vi "check syntax_core.vi"(8 "error in (no error)":errorcluster caption="에러 입력(에러 없음)", 11 "Script Line_gpio 입력":refnum<class "Script Line_gpio.lvclass">) -> (0 "error out":errorcluster caption="에러 출력", 3 "Script Line_gpio 출력":refnum<class "Script Line_gpio.lvclass">)   [LabVIEW 2020, in "Script Line_gpio.lvclass"]
uses:
  Script Line_gpio.lvclass
  Script Line/Script Line.lvclass/Script Line.ctl
  Script Line_gpio.lvclass/Script Line_gpio.ctl
  327cb276-063d-4ad0-890d-a8e0501d4965.vi
  Script Line/Accessors/Read parameter.vi
  Script Line/Accessors/Read parameter string index.vi
  <vilib>/Comparison/Equal/Equal Functor/Equal Functor.lvclass
  Script Line/Script Line.lvclass
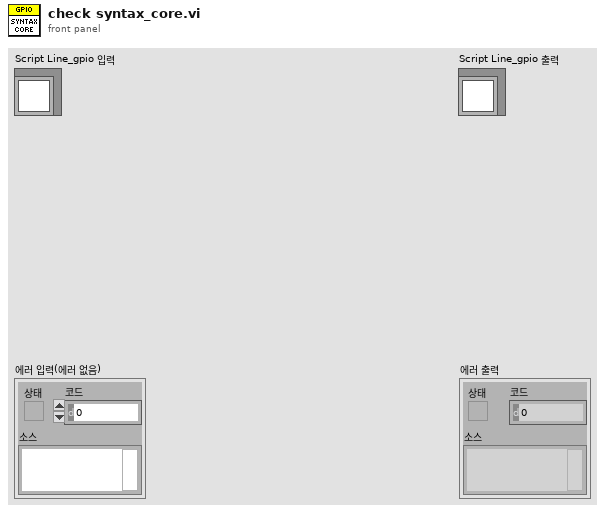
[diagram p1: front panel]
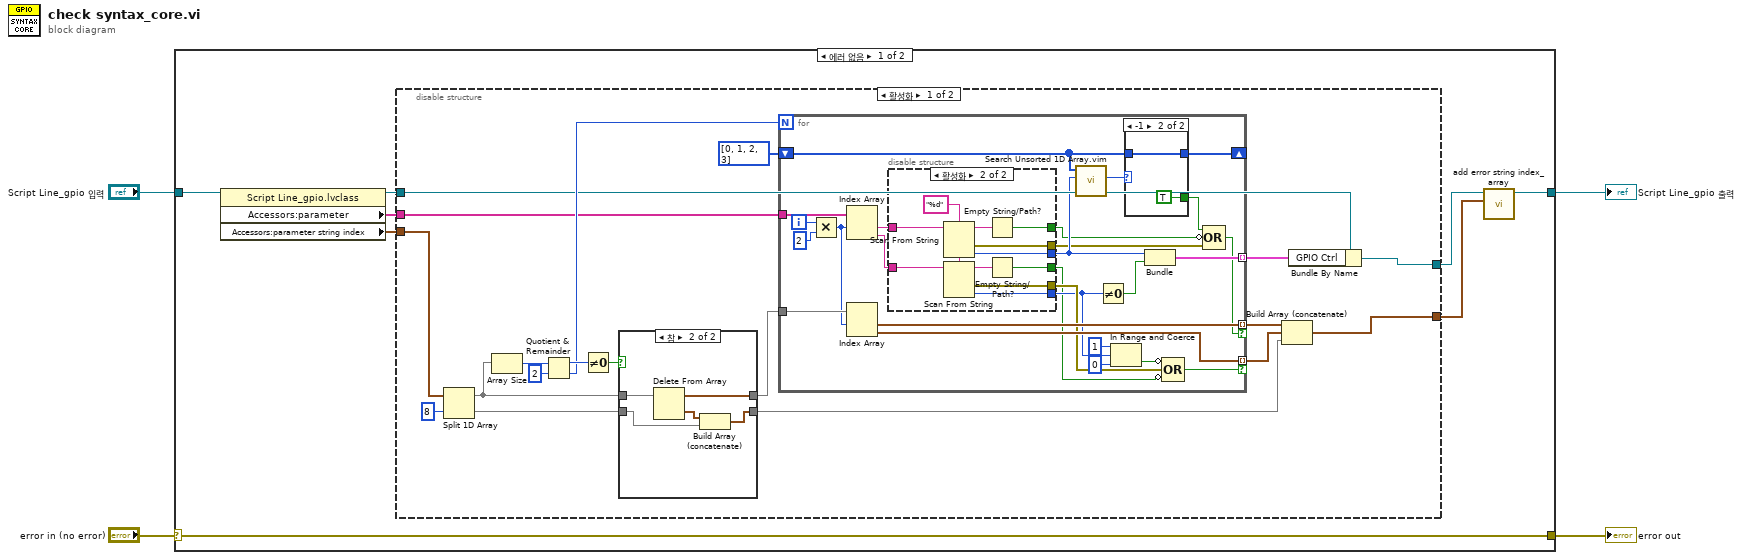
[diagram p0: block diagram]
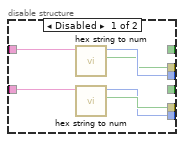
[diagram p2: hidden frame]
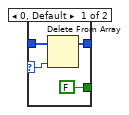
[diagram p3: hidden frame]
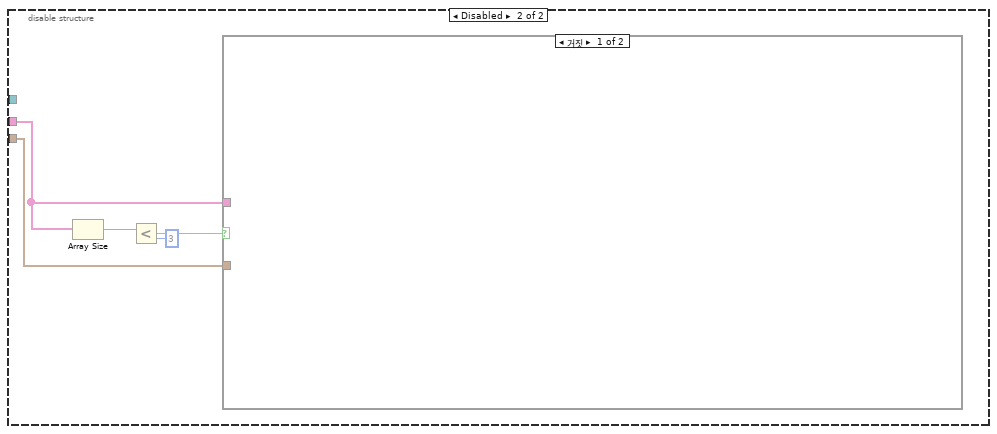
[diagram p5: hidden frame]
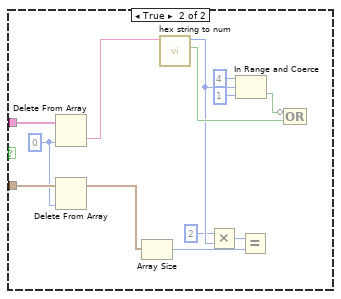
[diagram p6: hidden frame]
diagram:
  n1 = case shown="에러 없음" "error in (no error)" {
    selector: "error in (no error)" -> [w12 w107]
    tunnel: [w12 w107] -> w4
    tunnel: [w9 w106] -> w3
    tunnel: "Script Line_gpio 입력" -> [w11 w106]
    frame No Error {
      n2 = property class="Script Line_gpio.lvclass"(reference=w11) -> (reference out=w6:refnum<class "Script Line_gpio.lvclass">, "Accessors:parameter"=w8:string[], "Accessors:parameter string index"=w10:cluster{"start":u32, "end":u32}[])  [unwired: 1 in, 1 out]
      n3 = disable-structure shown="활성화" {
        disable-tunnel: w10 -> [w31 w89]
        disable-tunnel: w8 -> [w22 w88]
        disable-tunnel: [w16 _] -> w7
        disable-tunnel: w6 -> [w15 _]
        disable-tunnel: [w13 _] -> w5
        frame Enabled {
          n4 = Split 1D Array(array=w31, index=8 ("인덱스")) -> (first subarray=w25:cluster{"start":u32, "end":u32}[], second subarray=w24:cluster{"start":u32, "end":u32}[])
          n5 = Array Size(array=w25) -> (size(s)=w29:i32)
          n6 = Quotient & Remainder(x=w29, y=2) -> (x-y*floor(x/y)=w27:i32, floor(x/y)=w23:i32)
          n7 = Not Equal To 0?(x=w27) -> (x != 0?=w26:bool)
          n8 = case shown="참" w26 {
            tunnel: w25 -> [w82 w87]
            tunnel: [w82 w86] -> w21
            tunnel: w24 -> [w81 w85]
            tunnel: [w81 w83] -> w17
            frame False {
            }
            frame True {
              n9 = Delete From Array(array=w87) -> (deleted portion=w84:cluster{"start":u32, "end":u32}, array with subset deleted=w86:cluster{"start":u32, "end":u32}[])  [unwired: 2 in]
              n10 = Build Array (concatenate)(w84, w85) -> (w83:cluster{"start":u32, "end":u32}[])
            }
          }
          n11 = for {
            N: w23 -> [_]
            tunnel: w22 -> [w57]
            tunnel: w21 -> [w52]
            tunnel: [w50] -> w19 mode=indexing if=w35
            tunnel: [w49] -> w18 mode=indexing if=w44
            shift-right: [w41] -> _
            shift-left: i32[] [0, 1, 2, 3] -> [w42]
            tunnel: [w38] -> w14 mode=indexing
            i -> [w56]
            n12 = Multiply(x=w56, y=2) -> (x*y=w51:i32)
            n13 = Index Array(array=w57, index #1=w51) -> (element #1=w54:string, element #2=w53:string)  [unwired: 1 in]
            n14 = Index Array(array=w52, index #1=w51) -> (element #1=w50:cluster{"start":u32, "end":u32}, element #2=w49:cluster{"start":u32, "end":u32})  [unwired: 1 in]
            n15 = disable-structure shown="활성화" {
              disable-tunnel: w54 -> [w63 w74]
              disable-tunnel: w53 -> [w62 w73]
              disable-tunnel: [w61 w68] -> w45
              disable-tunnel: [w60 w69] -> w40
              disable-tunnel: [w59 w71] -> w37
              disable-tunnel: [w58 w70] -> w36
              disable-tunnel: [_ w65] -> w33
              disable-tunnel: [_ w64] -> w32
              frame Disabled {
                n16 = call "hex string to num.vi"("string"=w63) -> ("error"=w58:bool, "num"=w59:u32)  [unwired: 7 in, 2 out]
                n17 = call "hex string to num.vi"("string"=w62) -> ("error"=w61:bool, "num"=w60:u32)  [unwired: 7 in, 2 out]
              }
              frame Enabled {
                w72 = "%d" ("포맷 문자열")
                n18 = Scan From String(format string=w72, input string=w74) -> (remaining string=w67:string, error out=w70:errorcluster, output 1=w71:i32)  [unwired: 3 in, 1 out]
                n19 = Scan From String(format string=w72, input string=w73) -> (remaining string=w66:string, error out=w68:errorcluster, output 1=w69:i32)  [unwired: 3 in, 1 out]
                n20 = Empty String/Path?(string/path=w67) -> (empty?=w65:bool)
                n21 = Empty String/Path?(string/path=w66) -> (empty?=w64:bool)
              }
            }
            n22 = call "Search Unsorted 1D Array.vim"("element"=w37, "unsorted 1D array"=w42) -> ("index of element"=w43:i32)  [unwired: 9 in]
            n23 = Not Equal To 0?(x=w40) -> (x != 0?=w39:bool)
            n24 = In Range and Coerce(upper limit=u32 1 ("상위 리미트"), x=w40, lower limit=u32 0 ("하위 리미트")) -> (In Range?=w46:bool)  [unwired: 1 out]
            n25 = case shown="-1" w43 {
              selector: w43 -> [w77 _]
              tunnel: w42 -> [w78 w80]
              tunnel: [w76 w80] -> w41
              tunnel: [FALSE TRUE] -> w34
              frame 0, Default {
                n26 = Delete From Array(array=w78, index=w77) -> (array with subset deleted=w76:i32[])  [unwired: 1 in, 1 out]
              }
              frame -1 {
              }
            }
            n27 = Bundle(w37, w39) -> (w38:cluster{i32, bool})  [unwired: 1 in]
            n28 = Compound Arithmetic op=OR(invert w46, w45, invert w32) -> (w44:bool)
            n29 = Compound Arithmetic op=OR(w34, invert w33, w36) -> (w35:bool)
          }
          n30 = Build Array (concatenate)(w19, w18, w17) -> (w16:cluster{"start":u32, "end":u32}[])
          n31 = Bundle By Name(cluster=w15, "GPIO Ctrl"=w14) -> (w13:refnum<class "Script Line_gpio.lvclass">)
        }
        frame Disabled {
          n32 = Array Size(array=w88) -> (size(s)=w91:i32)
          n33 = Less?(x=w91, y=3) -> (x < y?=w90:bool)
          n34 = case shown="거짓" w90 {
            tunnel: w89 -> [_ w102]
            tunnel: w88 -> [_ w105]
            frame False {
            }
            frame True {
              w94 = 0 ("인덱스")
              n35 = Delete From Array(array=w105, index=w94) -> (deleted portion=w93:string)  [unwired: 1 in, 1 out]
              n36 = Delete From Array(array=w102, index=w94) -> (array with subset deleted=w95:cluster{"start":u32, "end":u32}[])  [unwired: 1 in, 1 out]
              n37 = Array Size(array=w95) -> (size(s)=w97:i32)
              n38 = call "hex string to num.vi"("string"=w93) -> ("error"=w101:bool, "num"=w99:u32)  [unwired: 7 in, 2 out]
              n39 = Multiply(x=u32 2 ("y"), y=w99) -> (x*y=w96:u32)
              n40 = In Range and Coerce(upper limit=u32 4 ("상위 리미트"), x=w99, lower limit=u32 1 ("하위 리미트")) -> (In Range?=w100:bool)  [unwired: 1 out]
              n41 = Equal?(x=w96, y=w97) -> ()  [unwired: 1 out]
              n42 = Compound Arithmetic op=OR(invert w100, w101) -> ()  [unwired: 1 out]
            }
          }
        }
      }
      n43 = call "add error string index_array.vi"("index_array"=w7, "Script Line 입력"=w5) -> ("Script Line 출력"=w9:refnum<class "Script Line_gpio.lvclass">)  [unwired: 8 in, 1 out]
    }
    frame Error {
    }
  }
  "error out" <- w4
  "Script Line_gpio 출력" <- w3
